vi "ALR messageB.vi"(5 "object":string="AZ1", 7 "date/time string":string, 8 "error in (no error)":errorcluster, 9 "ALRNames":refnum<data-value>, 10 "Alr_state":T1, 11 "ALR_msg":refnum<queue>) -> (0 "error out":errorcluster, 3 "new alr":bool)   [LabVIEW 2019, in "Alarms.lvlib"]
uses:
  Alarms.lvlib
  Ctl/ALRs_State.ctl
  Logik/Logik.lvlib
  Database/PostgreSQL.lvlib
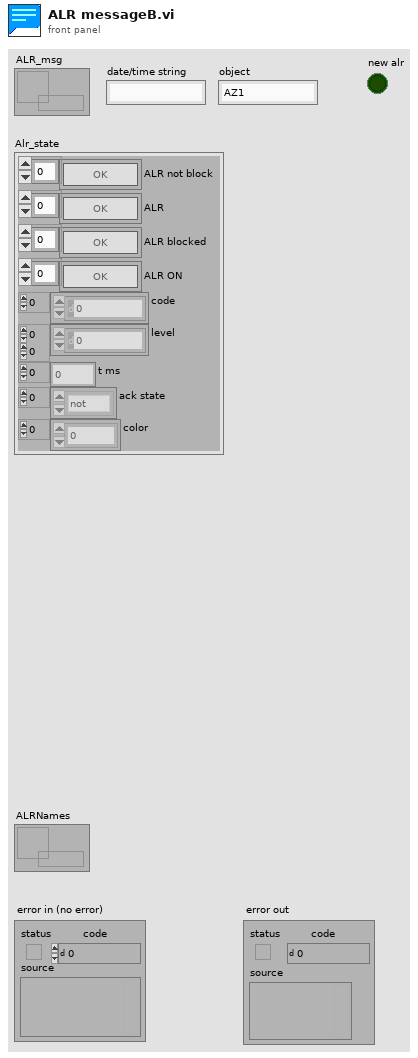
[diagram p1: front panel]
types:
  T1 = typedef "Alarms.lvlib/ALRs_State.ctl" = cluster{"ALR not block":bool[], "ALR":bool[], "ALR blocked":bool[], "ALR ON":bool[], "code":i32[], "level":i32[][], "t ms":u32[], "ack state":enum32{"not", "tripped", "reset", "ack"}[], "color":u32[]}
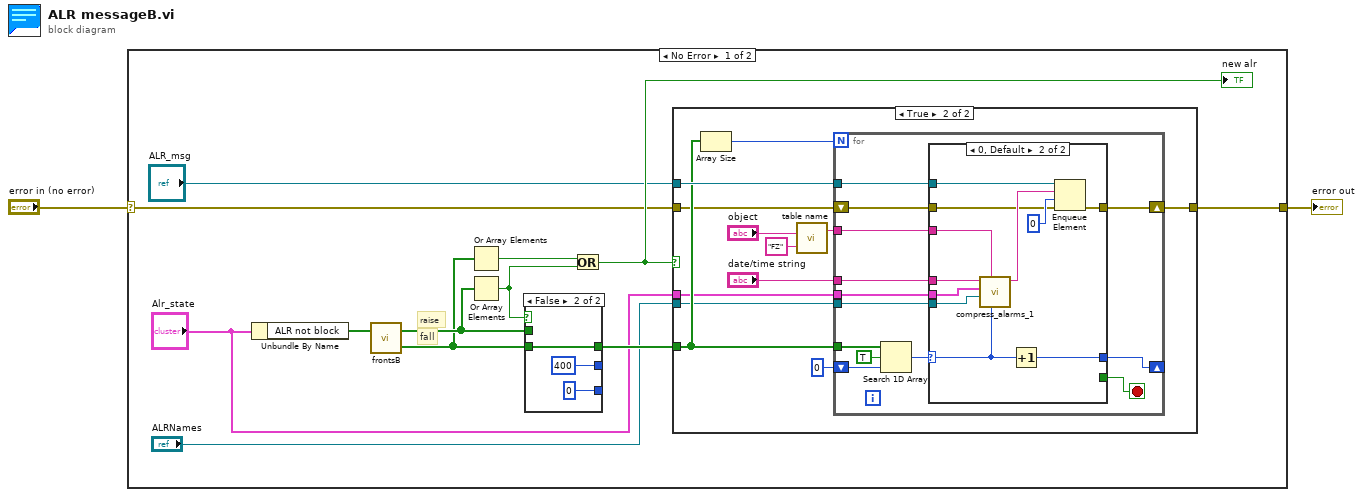
[diagram p0: block diagram]
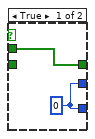
[diagram p2: hidden frame]
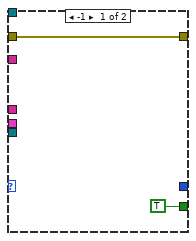
[diagram p4: hidden frame]
diagram:
  n1 = case shown="No Error" "error in (no error)" {
    selector: "error in (no error)" -> [w3 w59]
    tunnel: [w9 w59] -> w1
    frame No Error {
      # "fall"
      # "raise"
      n2 = Unbundle By Name("Alr_state") -> ("ALR not block"=w7:bool[])
      n3 = call "frontsB.vi"("IN"=w7) -> ("FALL"=w12:bool[], "RAISE"=w13:bool[])  [unwired: 1 in]
      n4 = Or Array Elements(Boolean array=w12) -> (logical OR=w10:bool)
      n5 = Or Array Elements(Boolean array=w13) -> (logical OR=w11:bool)
      n6 = case shown="False" w11 {
        tunnel: w13 -> [w16 _]
        tunnel: w12 -> [_ w19]
        tunnel: [w16 w19] -> w14
        tunnel: [w15 400 ("y")] -> _
        tunnel: [w15 0 ("y")] -> _
        frame True {
          w15 = 0 ("y")
        }
        frame False {
        }
      }
      n7 = Or(x=w10, y=w11) -> (x .or. y?=w5:bool)
      "new alr" <- w5
      n8 = case shown="True" w5 {
        tunnel: w14 -> [_ w30]
        tunnel: "ALR_msg" -> [_ w32]
        tunnel: w3 -> [w20 w27]
        tunnel: [w20 w21] -> w9
        tunnel: "Alr_state" -> [_ w26]
        tunnel: "ALRNames" -> [_ w25]
        frame False {
        }
        frame True {
          n9 = Array Size(array=w30) -> (size(s)=w31:i32)
          n10 = call "table name.vi"("postfix"="FZ", "object name"="object") -> ("table name"=w22:string)  [unwired: 1 in]
          n11 = for {
            N: w31 -> [_]
            tunnel: w30 -> [w45]
            tunnel: w32 -> [w42]
            shift-right: [w41] -> _
            shift-left: 0 -> [w40]
            tunnel: "date/time string" -> [w38]
            tunnel: w26 -> [w35]
            tunnel: w25 -> [w34]
            tunnel: w22 -> [w33]
            shift-right: [w36] -> w21
            shift-left: w27 -> [w37]
            stop <- w39 stop-if-true
            n12 = Search 1D Array(1D array=w45, element=TRUE, start index (0)=w40) -> (index of element=w43:i32)
            n13 = case shown="0, Default" w43 {
              selector: w43 -> [_ w58]
              tunnel: w42 -> [_ w56]
              tunnel: [_ w57] -> w41
              tunnel: [TRUE _] -> w39
              tunnel: w33 -> [_ w51]
              tunnel: w38 -> [_ w50]
              tunnel: w37 -> [w46 w53]
              tunnel: [w46 w52] -> w36
              tunnel: w35 -> [_ w49]
              tunnel: w34 -> [_ w48]
              frame -1 {
              }
              frame 0, Default {
                n14 = call "compress_alarms_1.vi"("N alr"=w58, "table"=w51, "ALRNames"=w48, "Alr_state"=w49, "date/time string"=w50) -> ("parameters"=w55:string)  [unwired: 6 in]
                n15 = Increment(x=w58) -> (x+1=w57:i32)
                n16 = Enqueue Element(queue=w56, element=w55, timeout in ms (-1)=0, error in (no error)=w53) -> (error out=w52:errorcluster)  [unwired: 2 out]
              }
            }
          }
        }
      }
    }
    frame Error {
    }
  }
  "error out" <- w1
